vi "Get Lockin Sweep Data.vi"(8 "error in (no error)":errorcluster, 10 "Channel":i32, 11 "MeasurementSMO in":refnum<class "AFM_Litho_Plugin.IV.lvclass">) -> (0 "error out":errorcluster, 1 "Sweep_AI":waveform(dbl)[](array[waveform]), 2 "Sweep_AO":waveform(dbl)[](array[waveform]), 3 "MeasurementSMO out":refnum<class "AFM_Litho_Plugin.IV.lvclass">)   [LabVIEW 2019, in "AFM_Litho_Plugin.IV.lvclass"]
uses:
  AFM_Litho_Plugin.IV.lvclass
  AFM_Litho_Plugin.IV.lvclass/AFM_Litho_Plugin.IV.ctl
  <userlib>/LevyLab/Lockin-Multichannel/Instrument.Lockin/Instrument.Lockin.lvclass
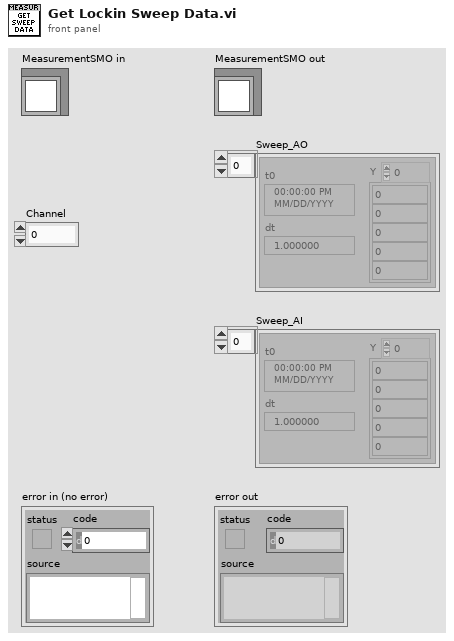
[diagram p1: front panel]
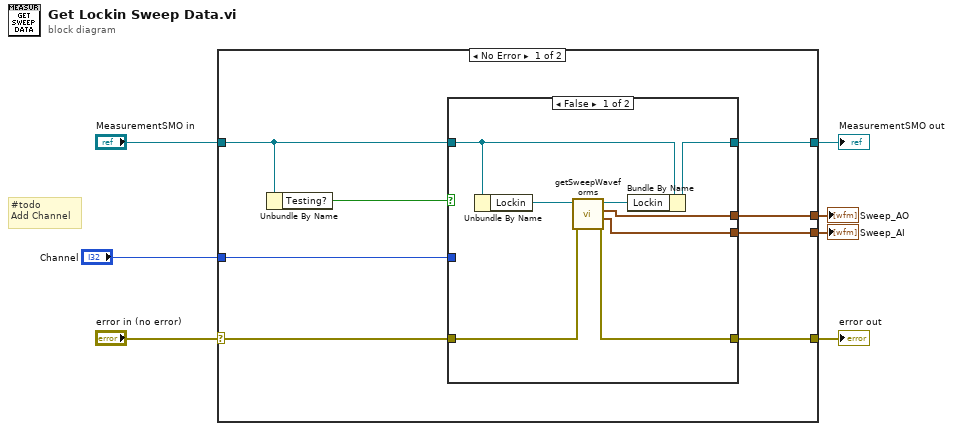
[diagram p0: block diagram]
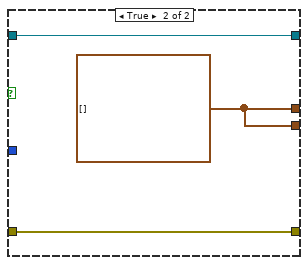
[diagram p2: hidden frame]
diagram:
  # "#todo\nAdd Channel"
  n1 = case shown="No Error" "error in (no error)" {
    selector: "error in (no error)" -> [w14 w28]
    tunnel: [w13 w28] -> w6
    tunnel: [w11 w27] -> w4
    tunnel: "MeasurementSMO in" -> [w12 w27]
    tunnel: [w10 _] -> w3
    tunnel: [w9 _] -> w2
    tunnel: "Channel" -> [w8 _]
    frame No Error {
      n2 = Unbundle By Name(w12) -> ("Testing?"=w15:bool)
      n3 = case shown="False" w15 {
        tunnel: w14 -> [w23 w25]
        tunnel: [w22 w25] -> w13
        tunnel: w12 -> [w20 w26]
        tunnel: [w19 w26] -> w11
        tunnel: [w17 w24] -> w10
        tunnel: [w16 w24] -> w9
        tunnel: w8 -> [_ _]
        frame False {
          n4 = Unbundle By Name(w20) -> ("Lockin"=w21:refnum<class "Instrument.Lockin.lvclass">)
          n5 = call <userlib>:"getSweepWaveforms.vi"("error in (no error)"=w23, "Instrument.Lockin in"=w21) -> ("error out"=w22:errorcluster, "Sweep_AI"=w16:waveform(dbl)[], "Sweep_AO"=w17:waveform(dbl)[], "Instrument.Lockin out"=w18:refnum<class "Instrument.Lockin.lvclass">)  [unwired: 6 in]
          n6 = Bundle By Name(cluster=w20, "Lockin"=w18) -> (w19:refnum<class "AFM_Litho_Plugin.IV.lvclass">)
        }
        frame True {
          w24 = waveform(dbl)[] [] ("Sweep_AO")
        }
      }
    }
    frame Error {
    }
  }
  "error out" <- w6
  "MeasurementSMO out" <- w4
  "Sweep_AO" <- w3
  "Sweep_AI" <- w2
